vi "SOAE-Delete Last File.vi"(0 "State":T1, 1 "XYGraph in":refnum<vi>, 2 "Listbox":refnum<vi>) -> (4 "State out":T1, 15 "error out":errorcluster)   [LabVIEW 2020]
uses:
  Typedefs/SOAE-State.ctl
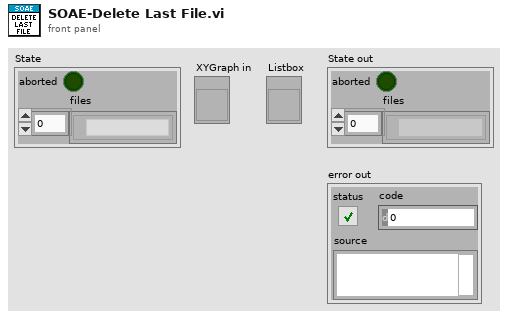
[diagram p1: front panel]
types:
  T1 = typedef "SOAE-State.ctl" = cluster{"aborted":bool, "files":path[]}
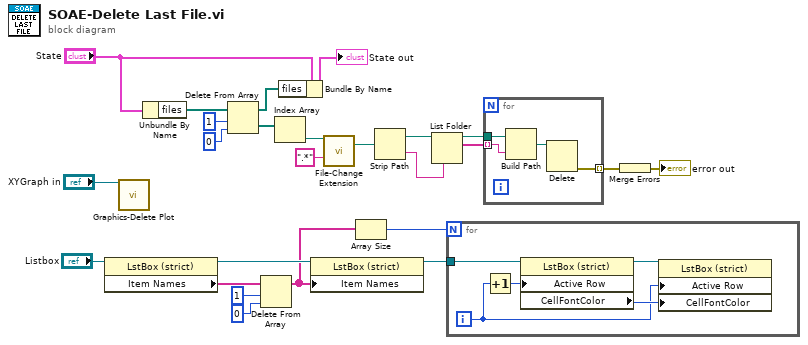
[diagram p0: block diagram]
diagram:
  n1 = property class="LstBox (strict)"(reference="Listbox") -> (reference out=w4:refnum<vi>, "Item Names"=w7:string[])  [unwired: 1 in, 1 out]
  n2 = call "Graphics-Delete Plot.vi"("XYGraph in"="XYGraph in") -> ()  [unwired: 13 in, 2 out]
  n3 = Unbundle By Name("State") -> ("files"=w24:path[])
  n4 = Delete From Array(array=w24, length=1, index=0) -> (deleted portion=w21:path[], array with subset deleted=w19:path[])
  n5 = Delete From Array(array=w7, length=1, index=0) -> (array with subset deleted=w3:string[])  [unwired: 1 out]
  n6 = Index Array(array=w21) -> (element=w18:path)  [unwired: 1 in]
  n7 = Bundle By Name(cluster="State", "files"=w19) -> (→"State out":T1)
  n8 = property class="LstBox (strict)"(reference=w4, "Item Names"=w3) -> (reference out=w1:refnum<vi>)  [unwired: 1 in, 1 out]
  n9 = call "File-Change Extension.vi"("Path"=w18, "new extension"=".*") -> ("new path"=w16:path)  [unwired: 13 in]
  n10 = Array Size(array=w3) -> (size(s)=w2:i32)
  n11 = Strip Path(path=w16) -> (stripped path=w15:path, name=w14:string)
  n12 = List Folder(path=w15, pattern=w14) -> (path out=w13:path, filenames=w12:string[])  [unwired: 2 in, 2 out]
  n13 = for {
    N: w2 -> [_]
    tunnel: w1 -> [w30]
    i -> [w26]
    n14 = Increment(x=w26) -> (x+1=w27:i32)
    n15 = property class="LstBox (strict)"(reference=w30, "Active Row"=w27) -> (reference out=w29:refnum<vi>, "CellFontColor"=w28:u32)  [unwired: 1 in, 1 out]
    n16 = property class="LstBox (strict)"(reference=w29, "Active Row"=w26, "CellFontColor"=w28) -> ()  [unwired: 1 in, 2 out]
  }
  n17 = for {
    tunnel: w13 -> [w34]
    tunnel: w12 -> [w33] mode=indexing
    tunnel: [w31] -> w11 mode=indexing
    n18 = Build Path(base path=w34, name or relative path=w33) -> (appended path=w32:path)
    n19 = Delete(path (use dialog)=w32) -> (error out=w31:errorcluster)  [unwired: 4 in, 2 out]
  }
  n20 = Merge Errors(w11) -> (→"error out":errorcluster)
